vi "sub_ofdm_simple_delayed_mult_CFO_sync_single.vi"(8 "CP length":i32=64, 9 "FFT size":i32=256, 11 "time samples":cdb[](array[numeric])) -> (3 "sync ofdm symbol":cdb[](array[numeric]))   [LabVIEW 2014]
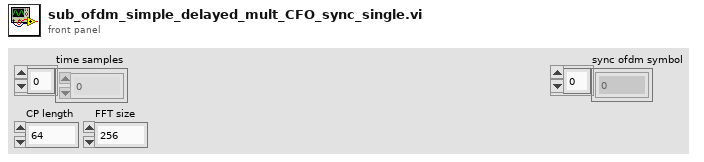
[diagram p1: front panel]
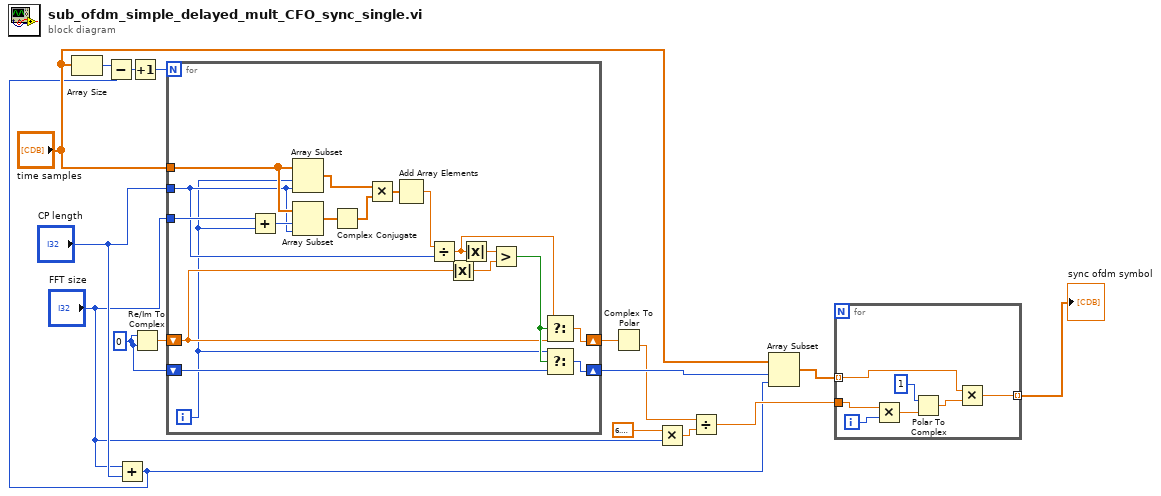
[diagram p0: block diagram]
diagram:
  w14 = 0
  n1 = Array Size(array="time samples") -> (size(s)=w16:i32)
  n2 = Add(x="FFT size", y="CP length") -> (x+y=w2:i32)
  n3 = Subtract(x=w16, y=w2) -> (x-y=w17:i32)
  n4 = Increment(x=w17) -> (x+1=w1:i32)
  n5 = Re/Im To Complex(1:w14, 2:w14) -> (0:w15:cdb)
  n6 = for {
    N: w1 -> [_]
    tunnel: "CP length" -> [w27]
    tunnel: "time samples" -> [w35]
    tunnel: "FFT size" -> [w28]
    shift-right: [w18] -> w11
    shift-left: w15 -> [w21]
    shift-right: [w22] -> w13
    shift-left: w14 -> [w23]
    i -> [w19]
    n7 = Add(x=w28, y=w19) -> (x+y=w34:i32)
    n8 = Array Subset(array=w35, index=w19, length=w27) -> (w32:cdb[])
    n9 = Array Subset(array=w35, index=w34, length=w27) -> (w33:cdb[])
    n10 = Complex Conjugate(1:w33) -> (0:w31:cdb[])
    n11 = Multiply(x=w32, y=w31) -> (x*y=w30:cdb[])
    n12 = Add Array Elements(numeric array=w30) -> (sum=w29:cdb)
    n13 = Divide(x=w29, y=w27) -> (x/y=w20:cdb)
    n14 = Absolute Value(x=w21) -> (abs(x)=w25:dbl)
    n15 = Absolute Value(x=w20) -> (abs(x)=w26:dbl)
    n16 = Greater?(x=w26, y=w25) -> (0:w24:bool)
    n17 = Select(t=w20, s=w24, f=w21) -> (s? t:f=w18:cdb)
    n18 = Select(t=w19, s=w24, f=w23) -> (s? t:f=w22:i32)
  }
  n19 = Complex To Polar(r * e^(i*theta)=w11) -> (theta=w7:dbl)  [unwired: 1 out]
  n20 = Multiply(x=6.283185307179586, y="FFT size") -> (x*y=w8:dbl)
  n21 = Divide(x=w7, y=w8) -> (x/y=w6:dbl)
  n22 = Array Subset(array="time samples", index=w13, length=w2) -> (w10:cdb[])
  n23 = for {
    tunnel: w10 -> [w37] mode=indexing
    tunnel: w6 -> [w41]
    tunnel: [w36] -> w5 mode=indexing
    i -> [w42]
    n24 = Multiply(x=w41, y=w42) -> (x*y=w40:dbl)
    n25 = Polar To Complex(1:w40, 2:1) -> (0:w38:cdb)
    n26 = Multiply(x=w37, y=w38) -> (x*y=w36:cdb)
  }
  "sync ofdm symbol" <- w5
